vi "ParseDataTypeToString.vi"(1 "Variant":variant, 5 "error in (no error)":errorcluster) -> (15 "Name":string, 17 "String":string, 19 "error out":errorcluster)   [LabVIEW 2018, in "Python.lvclass"]
uses:
  Python.lvclass
  <vilib>/Utility/Data Type/NI_Data Type.lvlib
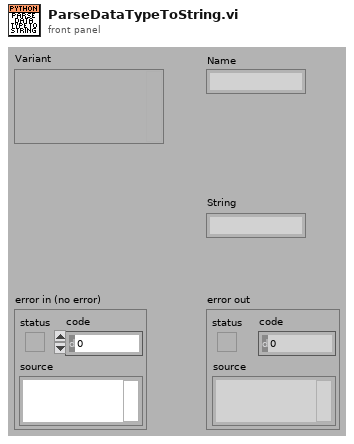
[diagram p1: front panel]
types:
  T1 = typedef "NI_Data Type.lvlib/Data Type.ctl" = enum8{"Invalid Type", "Void", "I8", "I16", "I32", "I64", "U8", "U16", "U32", "U64", "Single Float", "Double Float", "Extended Float", "Single Complex", "Double Complex", "Extended Complex", "Enum U8", "Enum U16", "Enum U32", "Enum U64", "Single Float With Unit", "Double Float With Unit", "Extended Float With Unit", "Single Complex with Unit", "Double Complex with Unit", "Extended Complex with Unit", "Boolean", "String", "Path", "Picture", "Tag", "Array", "Cluster", "Variant", "LV Variant", "Waveform", "Timestamp", "Digital Waveform", "Digital Data", "ExpressData", "Refnum", "External Data", "VI", "Poly VI", "LabVIEW Class Instance", "Fixed Point"}
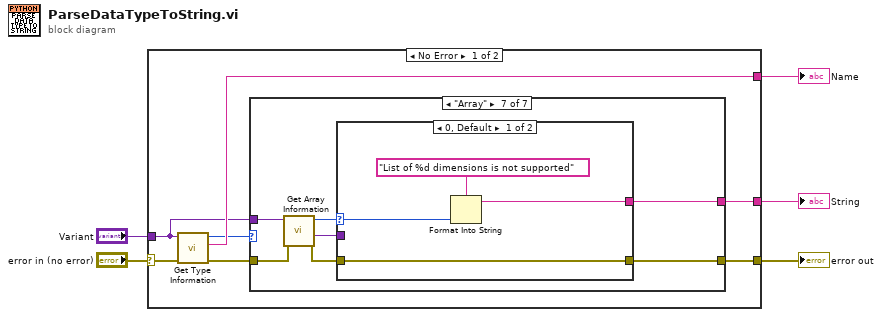
[diagram p0: block diagram]
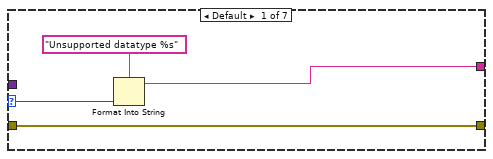
[diagram p2: hidden frame]
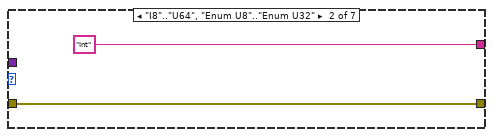
[diagram p3: hidden frame]
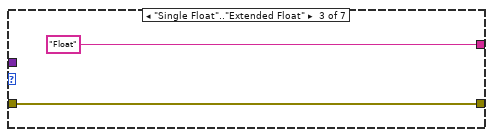
[diagram p4: hidden frame]
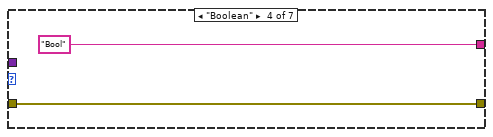
[diagram p5: hidden frame]
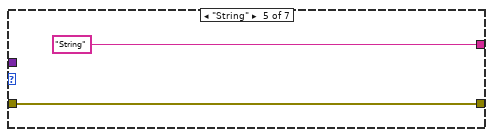
[diagram p6: hidden frame]
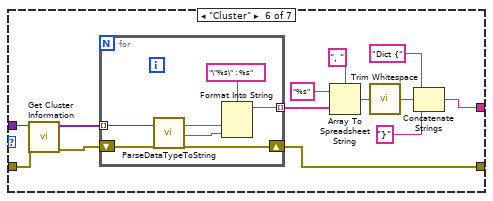
[diagram p7: hidden frame]
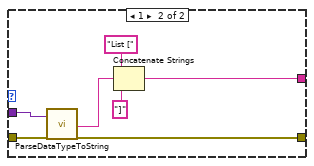
[diagram p8: hidden frame]
diagram:
  n1 = case shown="No Error" "error in (no error)" {
    selector: "error in (no error)" -> [w7 w63]
    tunnel: [w6 w63] -> w4
    tunnel: "Variant" -> [w10 _]
    tunnel: [w12 _] -> w2
    tunnel: [w8 _] -> w1
    frame No Error {
      n2 = call <vilib>:"Get Type Information.vi"("error in (no error)"=w7, "Variant"=w10) -> ("error out"=w9:errorcluster, "Name"=w12:string, "Type"=w11:T1)  [unwired: 5 in, 2 out]
      n3 = case shown="\"Array\"" w11 {
        selector: w11 -> [w14 _ _ _ _ _ _]
        tunnel: [w13 "Int" "Float" "Bool" "String" w34 w51] -> w8
        tunnel: w10 -> [_ _ _ _ _ w37 w50]
        tunnel: w9 -> [w16 w17 w19 w21 w23 w27 w48]
        tunnel: [w16 w17 w19 w21 w23 w25 w46] -> w6
        frame Default {
          n4 = Format Into String(format string="Unsupported datatype %s", w14) -> (resulting string=w13:string)  [unwired: 2 in, 1 out]
        }
        frame "I8".."U64", "Enum U8".."Enum U32" {
        }
        frame "Single Float".."Extended Float" {
        }
        frame "Boolean" {
        }
        frame "String" {
        }
        frame "Cluster" {
          n5 = call <vilib>:"Get Cluster Information.vi"("error in (no error)"=w27, "Variant"=w37) -> ("error out"=w26:errorcluster, "Cluster Elements"=w36:variant[])  [unwired: 8 in]
          n6 = for {
            tunnel: w36 -> [w42] mode=indexing
            tunnel: [w43] -> w32 mode=indexing
            shift-right: [w38] -> w25
            shift-left: w26 -> [w39]
            n7 = call "ParseDataTypeToString.vi"("Variant"=w42, "error in (no error)"=w39) -> ("Name"=w41:string, "String"=w40:string, "error out"=w38:errorcluster)  [unwired: 15 in]
            n8 = Format Into String(format string="\"%s\" : %s", w41, w40) -> (resulting string=w43:string)  [unwired: 2 in, 1 out]
          }
          n9 = Array To Spreadsheet String(delimiter (Tab)=", ", array=w32, 3:"%s" ("format string")) -> (spreadsheet string=w29:string)
          n10 = call <vilib>:"Trim Whitespace.vi"("string"=w29) -> ("trimmed string"=w28:string)  [unwired: 1 in]
          n11 = Concatenate Strings("Dict {", w28, "}") -> (w34:string)
        }
        frame "Array" {
          n12 = call <vilib>:"Get Array Information.vi"("error in (no error)"=w48, "Variant"=w50) -> ("error out"=w47:errorcluster, "Array Element Data Type"=w49:variant, "Number of Dimensions"=w45:i32)  [unwired: 6 in, 1 out]
          n13 = case shown="0, Default" w45 {
            selector: w45 -> [w54 _]
            tunnel: [w52 w62] -> w51
            tunnel: w49 -> [_ w59]
            tunnel: w47 -> [w55 w57]
            tunnel: [w55 w56] -> w46
            frame 0, Default {
              n14 = Format Into String(format string="List of %d dimensions is not supported", w54) -> (resulting string=w52:string)  [unwired: 2 in, 1 out]
            }
            frame 1 {
              n15 = call "ParseDataTypeToString.vi"("Variant"=w59, "error in (no error)"=w57) -> ("String"=w58:string, "error out"=w56:errorcluster)  [unwired: 15 in, 1 out]
              n16 = Concatenate Strings("List [", w58, "]") -> (w62:string)
            }
          }
        }
      }
    }
    frame Error {
    }
  }
  "error out" <- w4
  "String" <- w1
  "Name" <- w2
